vi "LakeShore336_Controller.vi"() -> ()   [LabVIEW 2018]
uses:
  <instrlib>/Lake Shore 336/Public/Data/Sensor Data (Single Reading).vi
  <instrlib>/Lake Shore 336/Lake Shore 336.lvlib
panel:
  in  "Ramp Rate (0.0)":dbl=5.0 format="%.1f"
  out "Heater Status 2\nStage":u16(ring) items=["No Error", "Heater Open Load", "Heater Short"]
  out "Heater Status 1":u16(ring) items=["No Error", "Heater Open Load", "Heater Short"]
  in  "Instrument Setup?\nOff / On":bool
  out "Out4 Setpoint":dbl format="%.5f"
  out "Out3 Setpoint":dbl format="%.5f"
  out "Out2 Setpoint":dbl format="%.5f"
  out "Out1 Setpoint":dbl format="%.5f"
  in  "Output's Control Loop (1:1)\n1 - ?\n2 - Stage\n3 - ?\n4 - ?":u16(ring)=2 items=["1"=1, "2"=2, "3"=3, "4"=4]
  in  "Setpoint (0.00000)":dbl=294.0 format="%.5f"
  in  "Setpoint Ramping \nEnable (F: Off)":bool=TRUE
  in  "Sampling (Milliseconds)\nMin 1ms":u32=250
  in  "stop":bool
  out "Temp vs Vg : XYGraph":cluster{"Y":dbl[], "Y":dbl[]}[](graph)
  out "Temp vs Vg : TimeGraph":cluster{i32, "Sensor Data":dbl}[](graph)
  in  "Data Source (0:Kelvin)":u16(ring) items=["Kelvin", "Celsius", "Sensor Units"]
  in  "Input (0:A)\nA - Sample\nB - Rad Shield\nC - Arm\nD - Disabled":u16(ring) items=["A", "B", "C", "D"]
  in  "Serial Configuration 2":T1={"Baud Rate"=57600, "Parity"=1, "Data Bits"=7, "Stop Bits"=10, "Flow Control"=0} {"Flow Control" items=["None", "XON/XOFF", "RTS/CTS", "XON/XOFF & RTS/CTS", "DTR/DSR", "XON/XOFF & DTR/DSR"]; "Stop Bits" items=["1.0"=10, "1.5"=15, "2.0"=20]; "Data Bits" items=["7"=7, "8"=8]; "Parity" items=["None", "Odd", "Even", "Mark", "Space"]; "Baud Rate" items=["300"=300, "600"=600, "1200"=1200, "2400"=2400, "4800"=4800, "9600"=9600, "19200"=19200, "38400"=38400, "57600"=57600]}
  in  "LakeShore 336 esource name":refnum<visa-resource-name>="GPIB0::12::INSTR"
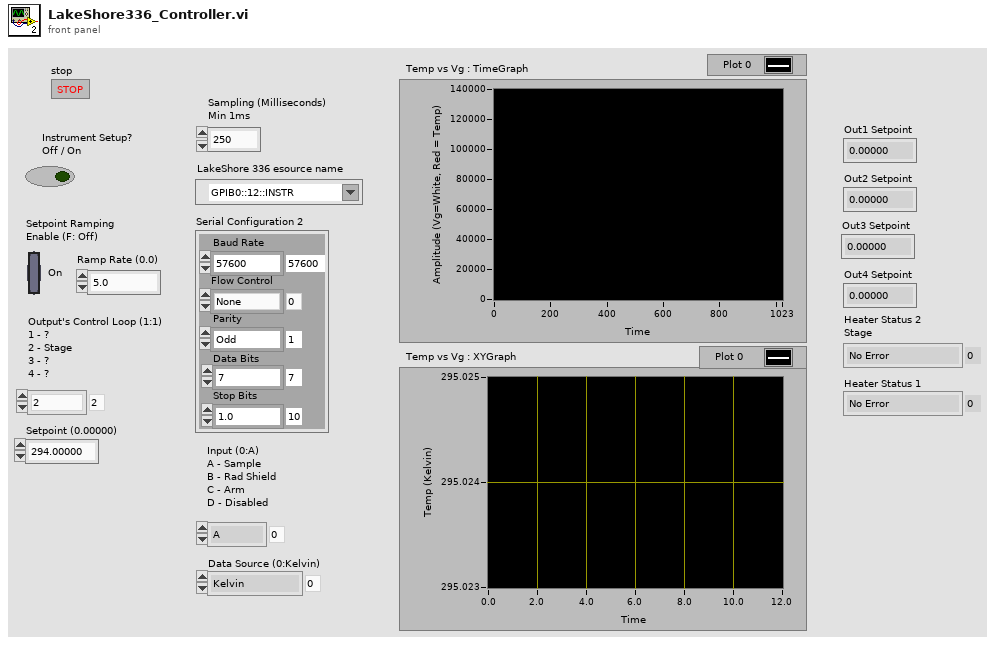
[diagram p1: front panel]
types:
  T1 = cluster{"Baud Rate":u32, "Parity":u16, "Data Bits":u16, "Stop Bits":u16, "Flow Control":u16}
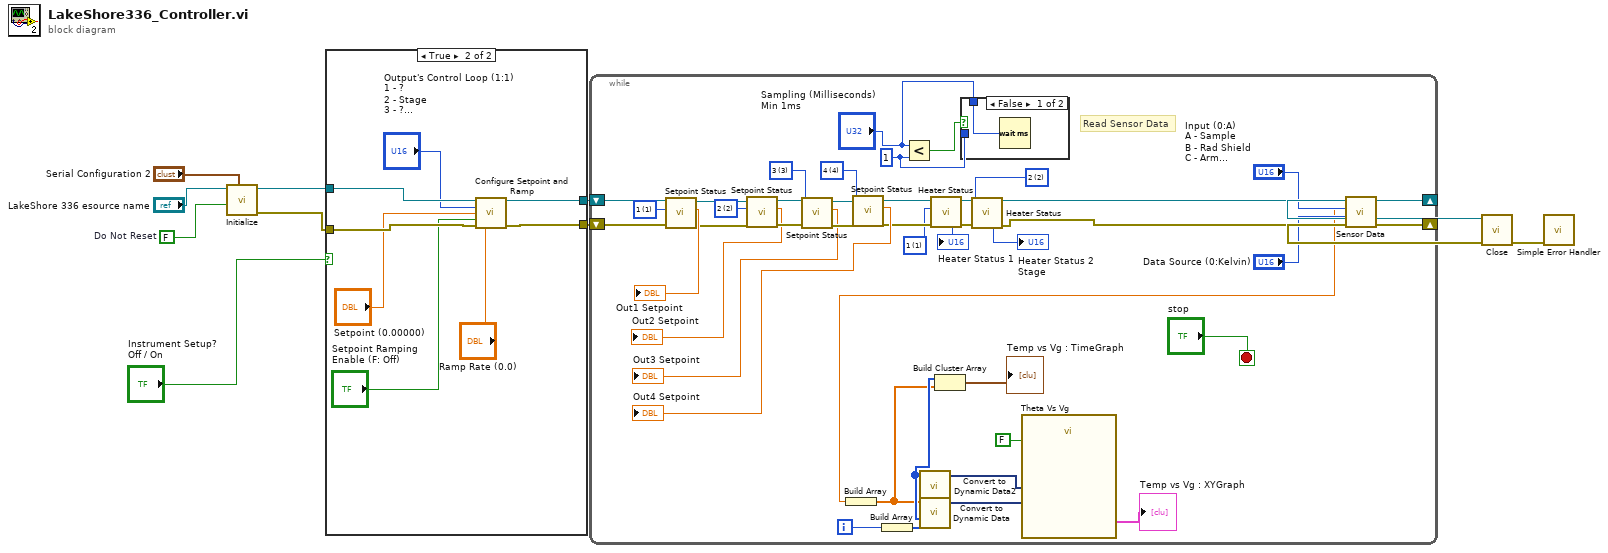
[diagram p0: block diagram]
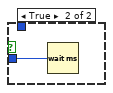
[diagram p3: hidden frame]
diagram:
  w9 = FALSE  # Do Not Reset
  n1 = call <instrlib>:"Initialize.vi"("Serial Configuration"="Serial Configuration 2", "Reset (True)"=w9, "VISA resource name"="LakeShore 336 esource name") -> ("error out"=w5:errorcluster, "VISA resource name out"=w3:refnum<visa-resource-name>)  [unwired: 7 in]
  n2 = case shown="True" "Instrument Setup?\nOff / On" {
    tunnel: w5 -> [w12 w21]
    tunnel: [w12 w20] -> w4
    tunnel: w3 -> [w13 w19]
    tunnel: [w13 w18] -> w2
    frame False {
    }
    frame True {
      n3 = call <instrlib>:"Configure Setpoint and Ramp.vi"("VISA resource name"=w19, "Output's Control Loop (1:1)"="Output's Control Loop (1:1)\n1 - ?\n2 - Stage\n3 - ?\n4 - ?", "Setpoint (0.00000)"="Setpoint (0.00000)", "Setpoint Ramping \nEnable (F: Off)"="Setpoint Ramping \nEnable (F: Off)", "error in (no error)"=w21, "Ramp Rate (0.0)"="Ramp Rate (0.0)") -> ("VISA resource name out"=w18:refnum<visa-resource-name>, "error out"=w20:errorcluster)  [unwired: 8 in]
    }
  }
  n4 = while {
    shift-right: [w62] -> w7
    shift-left: w2 -> [w46]
    shift-right: [w61] -> w6
    shift-left: w4 -> [w42]
    i -> [w54]
    stop <- "stop" stop-if-true
    w24 = u16 2 items=["1"=1, "2"=2] ("Heater Output (1:1)")
    w25 = u16 1 items=["1"=1, "2"=2] ("Heater Output (1:1)")
    w35 = u16 4 items=["1"=1, "2"=2, "3"=3, "4"=4] ("Output (1:1)")
    w36 = u16 3 items=["1"=1, "2"=2, "3"=3, "4"=4] ("Output (1:1)")
    w37 = u16 2 items=["1"=1, "2"=2, "3"=3, "4"=4] ("Output (1:1)")
    w38 = u16 1 items=["1"=1, "2"=2, "3"=3, "4"=4] ("Output (1:1)")
    w49 = u32 1 ("y")
    # "Read Sensor Data"
    n5 = call <instrlib>:"Setpoint Status.vi"("error in (no error)"=w42, "Output (1:1)"=w38, "VISA resource name"=w46) -> ("error out"=w41:errorcluster, "Setpoint"=→"Out1 Setpoint":dbl, "VISA resource name out"=w45:refnum<visa-resource-name>)  [unwired: 6 in]
    n6 = call <instrlib>:"Setpoint Status.vi"("error in (no error)"=w41, "Output (1:1)"=w37, "VISA resource name"=w45) -> ("error out"=w40:errorcluster, "Setpoint"=→"Out2 Setpoint":dbl, "VISA resource name out"=w44:refnum<visa-resource-name>)  [unwired: 6 in]
    n7 = call <instrlib>:"Setpoint Status.vi"("error in (no error)"=w40, "Output (1:1)"=w36, "VISA resource name"=w44) -> ("error out"=w39:errorcluster, "Setpoint"=→"Out3 Setpoint":dbl, "VISA resource name out"=w43:refnum<visa-resource-name>)  [unwired: 6 in]
    n8 = call <instrlib>:"Setpoint Status.vi"("error in (no error)"=w39, "Output (1:1)"=w35, "VISA resource name"=w43) -> ("error out"=w29:errorcluster, "Setpoint"=→"Out4 Setpoint":dbl, "VISA resource name out"=w27:refnum<visa-resource-name>)  [unwired: 6 in]
    n9 = Build Array(w54) -> (w52:i32[])
    n10 = Less?(x="Sampling (Milliseconds)\nMin 1ms", y=w49) -> (x < y?=w50:bool)
    n11 = call "Convert to Dynamic Data2"("Array"=w52) -> ("Dynamic Data Type"=w53:dynamicdata)  [unwired: 3 in]
    n12 = call <instrlib>:"Heater Status.vi"("error in (no error)"=w29, "Heater Output (1:1)"=w25, "VISA resource name"=w27) -> ("error out"=w28:errorcluster, "Heater Status"=→"Heater Status 1":u16, "VISA resource name out"=w26:refnum<visa-resource-name>)  [unwired: 6 in]
    n13 = case shown="False" w50 {
      tunnel: w49 -> [_ w66]
      tunnel: "Sampling (Milliseconds)\nMin 1ms" -> [w65 _]
      frame False {
        n14 = Wait (ms)(milliseconds to wait=w65) -> ()  [unwired: 1 out]
      }
      frame True {
        n15 = Wait (ms)(milliseconds to wait=w66) -> ()  [unwired: 1 out]
      }
    }
    n16 = call <instrlib>:"Heater Status.vi"("error in (no error)"=w28, "Heater Output (1:1)"=w24, "VISA resource name"=w26) -> ("error out"=w22:errorcluster, "Heater Status"=→"Heater Status 2\nStage":u16, "VISA resource name out"=w23:refnum<visa-resource-name>)  [unwired: 6 in]
    n17 = call-poly <instrlib>:"Sensor Data.vi"("error in (no error)"=w22, "Data Source (0:Kelvin)"="Data Source (0:Kelvin)", "Input (0:A)"="Input (0:A)\nA - Sample\nB - Rad Shield\nC - Arm\nD - Disabled", "VISA resource name"=w23) -> ("error out"=w61:errorcluster, "Sensor Data"=w56:dbl, "VISA resource name out"=w62:refnum<visa-resource-name>)  [unwired: 5 in]
    n18 = Build Array(w56) -> (w51:dbl[])
    n19 = call "Convert to Dynamic Data"("Array"=w51) -> ("Dynamic Data Type"=w55:dynamicdata)  [unwired: 3 in]
    n20 = Build Cluster Array(w52, w51) -> (→"Temp vs Vg : TimeGraph":cluster{i32, "Sensor Data":dbl}[])
    n21 = call "Theta Vs Vg"("Reset"=FALSE, "Y Input"=w55, "X Input"=w53) -> ("XY Graph"=→"Temp vs Vg : XYGraph":cluster{"X":dbl[], "Y":dbl[]}[])  [unwired: 7 in, 1 out]
  }
  n22 = call <instrlib>:"Close.vi"("error in (no error)"=w6, "VISA resource name"=w7) -> ("error out"=w10:errorcluster)  [unwired: 9 in]
  n23 = call <vilib>:"Simple Error Handler.vi"("error in (no error)"=w10) -> ()  [unwired: 4 in, 5 out]
